vi "State (SubVI).vi"(8 "error in (no error)":errorcluster, 11 "VISA Refnum in":refnum<visa-resource-name>) -> (0 "error out":errorcluster, 3 "read buffer":string)   [LabVIEW 2021]
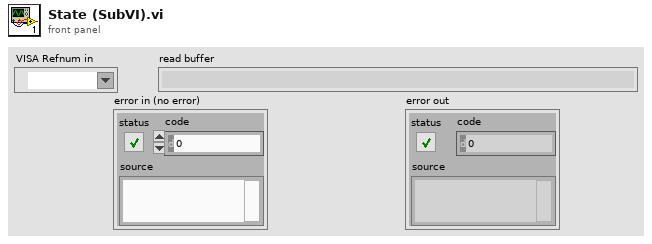
[diagram p1: front panel]
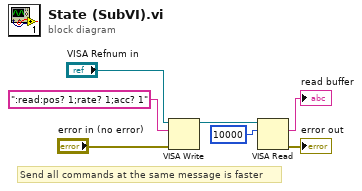
[diagram p0: block diagram]
diagram:
  # "Send all commands at the same message is faster"
  n1 = VISA Write(VISA resource name="VISA Refnum in", write buffer=":read:pos? 1;rate? 1;acc? 1", error in (no error)="error in (no error)") -> (VISA resource name out=w5:refnum<visa-resource-name>)  [unwired: 2 out]
  n2 = VISA Read(VISA resource name=w5, byte count=u32 10000) -> (read buffer=→"read buffer":string, error out=→"error out":errorcluster)  [unwired: 1 in, 2 out]
